vi "IntakeTeleop.vi"(10 "Outtake Button":bool, 11 "Intake Button":bool) -> ()   [LabVIEW 2017]
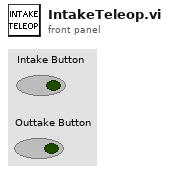
[diagram p1: front panel]
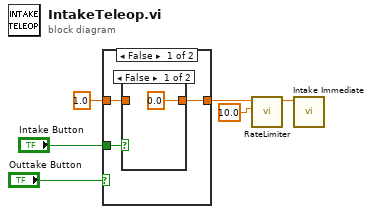
[diagram p0: block diagram]
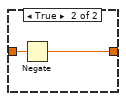
[diagram p3: hidden frame]
diagram:
  n1 = case shown="False" "Outtake Button" {
    tunnel: 1.0 -> [w7 w13]
    tunnel: [w8 w12] -> w3
    tunnel: "Intake Button" -> [w9 _]
    frame False {
      n2 = case shown="False" w9 {
        tunnel: [0.0 w11] -> w8
        tunnel: w7 -> [_ w11]
        frame False {
        }
        frame True {
        }
      }
    }
    frame True {
      n3 = Negate(x=w13) -> (-x=w12:dbl)
    }
  }
  n4 = call "RateLimiter.vi"("Max dx/dt"=10.0, "Input"=w3) -> ("Output"=w2:dbl)  [unwired: 9 in]
  n5 = call "Intake Immediate.vi"("Speed"=w2) -> ()  [unwired: 10 in, 1 out]
